vi "Add multiple rows.vi"(8 "error in (no error)":errorcluster, 10 "Row":string[][](array[string]), 11 "MulColLBTable.lvclass":refnum<class "MulColLBTable.lvclass">) -> (0 "error out":errorcluster, 3 "MulColLBTable.lvclass 2":refnum<class "MulColLBTable.lvclass">)   [LabVIEW 2020, in "MulColLBTable.lvclass"]
uses:
  MulColLBTable.lvclass
  MulColLBTable.lvclass/MulColLBTable.ctl
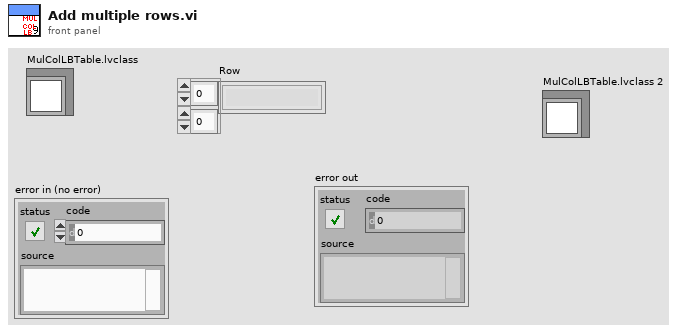
[diagram p1: front panel]
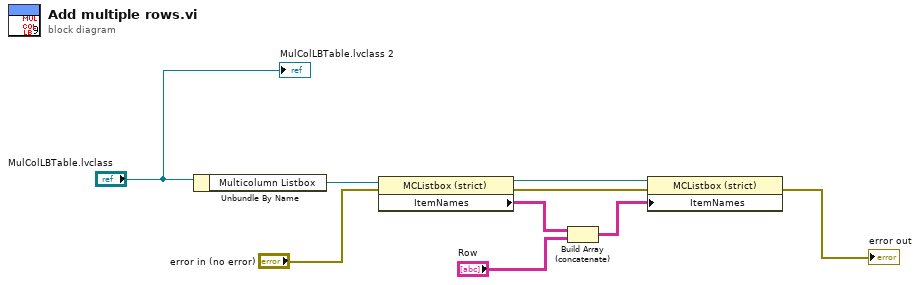
[diagram p0: block diagram]
diagram:
  n1 = Unbundle By Name("MulColLBTable.lvclass") -> ("Multicolumn Listbox"=w8:refnum<vi>)
  n2 = property class="MCListbox (strict)"(reference=w8, error in="error in (no error)") -> (reference out=w7:refnum<vi>, error out=w6:errorcluster, "ItemNames"=w3:string[][])
  n3 = Build Array (concatenate)(w3, "Row") -> (w2:string[][])
  n4 = property class="MCListbox (strict)"(reference=w7, error in=w6, "ItemNames"=w2) -> (error out=→"error out":errorcluster)  [unwired: 1 out]
  "MulColLBTable.lvclass 2" <- "MulColLBTable.lvclass"
